vi "Trigger Test.vi"() -> ()   [LabVIEW 2018]
panel:
  in  "Quit":bool
  out "Frames Per Second":dbl
  out "Image":u16[][](graph)
  out "Timestamp":dbl
  out "Error Out":errorcluster {"code" format="%.0x"}
  out "DCAM Version":string
  out "Library Version":string
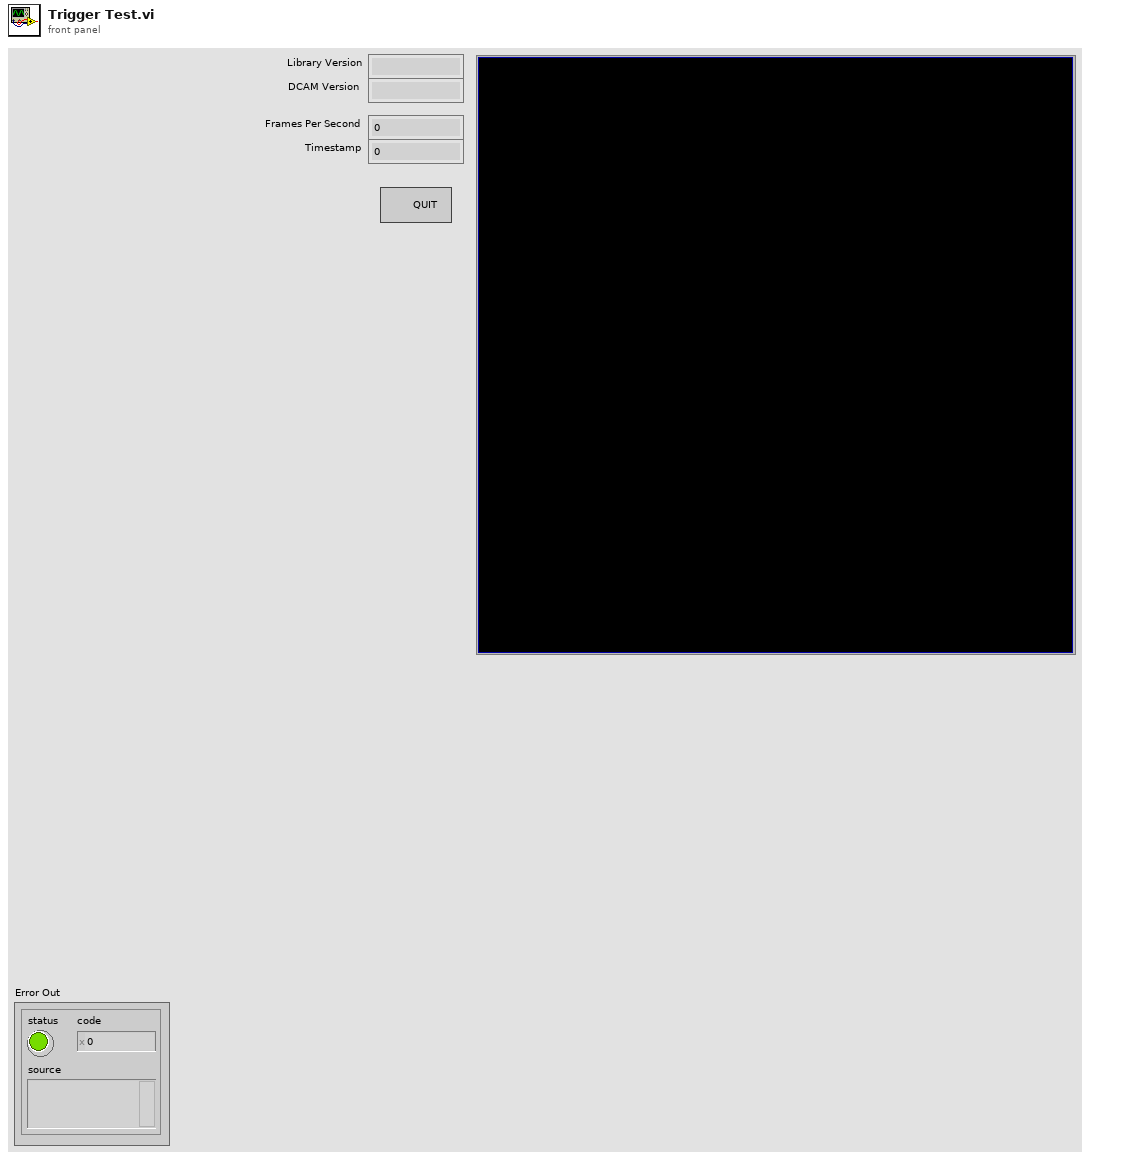
[diagram p1: front panel]
types:
  T1 = cluster{"Capture Library":string, "DCAM-API":string}
  T2 = cluster{"Horizontal Offset":i32, "Vertical Offset":i32, "Horizontal Size":i32, "Vertical Size":i32}
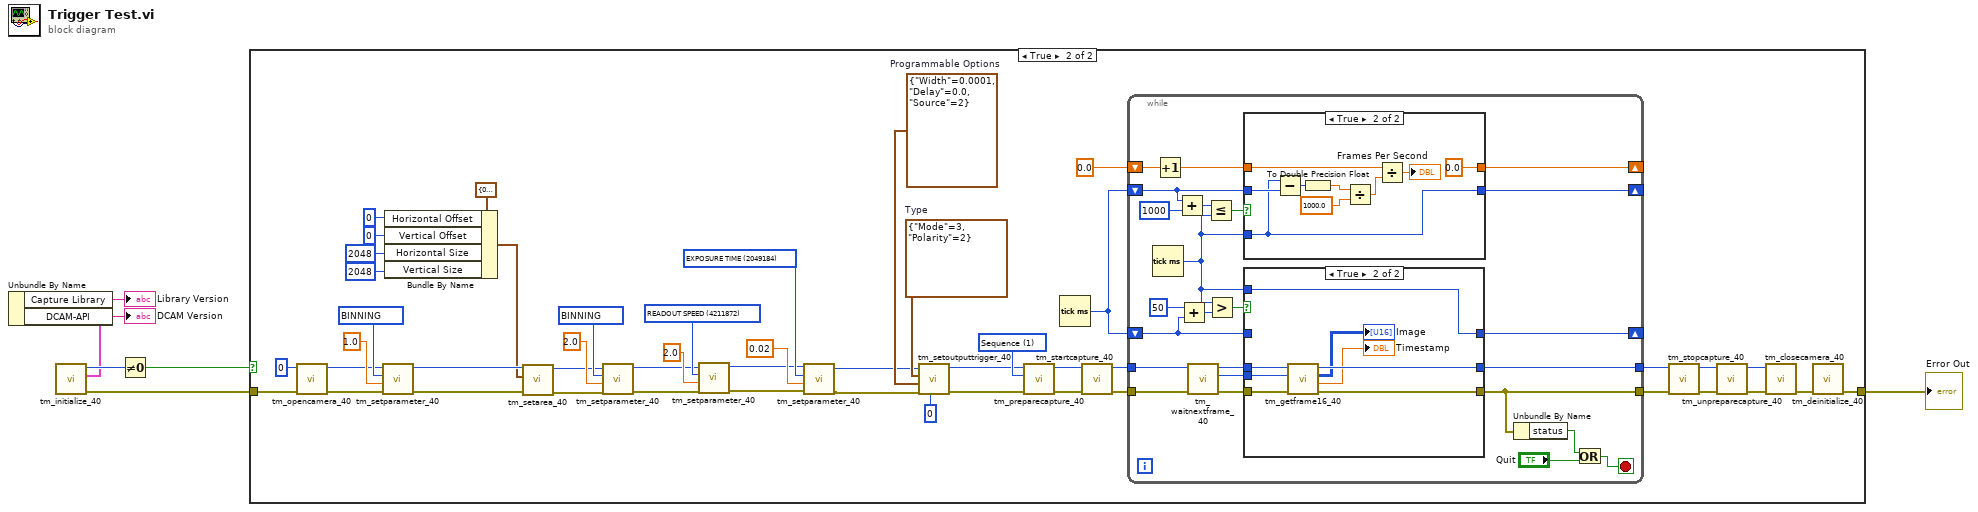
[diagram p0: block diagram]
diagram:
  n1 = call <userlib>:"tm_initialize_40.vi"() -> ("error out"=w2:errorcluster, "Version Info"=w6:T1, "Number Of Cameras"=w7:u32)  [unwired: 8 in, 1 out]
  n2 = Unbundle By Name(w6) -> ("Capture Library"=→"Library Version":string, "DCAM-API"=→"DCAM Version":string)
  n3 = Not Equal To 0?(x=w7) -> (x != 0?=w1:bool)
  n4 = case shown="True" w1 {
    tunnel: w2 -> [w8 w56]
    tunnel: [w8 w40] -> w3
    frame False {
    }
    frame True {
      w11 = cluster{"Width":dbl, "Delay":dbl, "Source":u32} {"Width"=0.0001, "Delay"=0.0, "Source"=2}  # Programmable Options
      w13 = cluster{"Mode":u32, "Polarity":u32} {"Mode"=3, "Polarity"=2}  # Type
      w19 = u32 2049184 items=["SENSOR MODE"=4212128, "READOUT SPEED"=4211872, "READOUT DIRECTION"=4211904, "BIT PER CHANNEL"=4342976, "TRIGGER GLOBAL EXPOSURE"=2049680, "TRIGGER DELAY"=1066480, "SYNC READOUT SYSTEM BLANK"=1066528, "SENSOR COOLER STATUS"=2115280, "EXPOSURE TIME"=2049184, "DEFECT CORRECT MODE"=4670368, "BINNING"=4215968, "TIMING READOUT TIME"=4223904, "INTERNAL FRAME RATE"=4225952, "INTERNAL FRAME INTERVAL"=4225968, "INTERNAL LINE SPEED"=4226000, "INTERNAL LINE INTERVAL"=4226016, "IMAGE WIDTH"=4343200, "IMAGE HEIGHT"=4343216, "IMAGE ROWBYTES"=4343232, "IMAGE FRAMEBYTES"=4343248, "IMAGE PIXEL TYPE"=4343296, "NUMBER OF OUTPUT TRIGGER CONNECTOR"=1852320, "OUTPUT TRIGGER SOURCE[0]"=1852576, "OUTPUT TRIGGER SOURCE[1]"=1852832, "OUTPUT TRIGGER SOURCE[2]"=1853088, "OUTPUT TRIGGER POLARITY[0]"=1852592, "OUTPUT TRIGGER POLARITY[1]"=1852848, "OUTPUT TRIGGER POLARITY[2]"=1853104, "OUTPUT TRIGGER ACTIVE[0]"=1852608, "OUTPUT TRIGGER ACTIVE[1]"=1852864, "OUTPUT TRIGGER ACTIVE[2]"=1853120, "OUTPUT TRIGGER DELAY[0]"=1852624, "OUTPUT TRIGGER DELAY[1]"=1852880, "OUTPUT TRIGGER DELAY[2]"=1853136, "OUTPUT TRIGGER PERIOD[0]"=1852640, "OUTPUT TRIGGER PERIOD[1]"=1852896, "OUTPUT TRIGGER PERIOD[2]"=1853152, "OUTPUT TRIGGER KIND[0]"=1852656, "OUTPUT TRIGGER KIND[1]"=1852912, "OUTPUT TRIGGER KIND[2]"=1853168, "OUTPUT TRIGGER PRE HSYNC COUNT"=1852704] ("Parameter")
      w25 = u32 4215968 items=["SENSOR MODE"=4212128, "READOUT SPEED"=4211872, "READOUT DIRECTION"=4211904, "TRIGGER GLOBAL EXPOSURE"=2049680, "TRIGGER DELAY"=1066480, "INTERNAL TRIGGER HANDLING"=1066496, "SYNC READOUT SYSTEM BLANK"=1066528, "SENSOR TEMPERATURE"=2115232, "SENSOR COOLER STATUS"=2115280, "EXPOSURE TIME"=2049184, "DEFECT CORRECT MODE"=4670368, "BINNING"=4215968, "INTERNAL LINE SPEED"=4226000, "INTERNAL LINE INTERVAL"=4226016, "NUMBER OF OUTPUT TRIGGER CONNECTOR"=1852320, "OUTPUT TRIGGER SOURCE[0]"=1852576, "OUTPUT TRIGGER SOURCE[1]"=1852832, "OUTPUT TRIGGER SOURCE[2]"=1853088, "OUTPUT TRIGGER POLARITY[0]"=1852592, "OUTPUT TRIGGER POLARITY[1]"=1852848, "OUTPUT TRIGGER POLARITY[2]"=1853104, "OUTPUT TRIGGER ACTIVE[0]"=1852608, "OUTPUT TRIGGER ACTIVE[1]"=1852864, "OUTPUT TRIGGER ACTIVE[2]"=1853120, "OUTPUT TRIGGER DELAY[0]"=1852624, "OUTPUT TRIGGER DELAY[1]"=1852880, "OUTPUT TRIGGER DELAY[2]"=1853136, "OUTPUT TRIGGER PERIOD[0]"=1852640, "OUTPUT TRIGGER PERIOD[1]"=1852896, "OUTPUT TRIGGER PERIOD[2]"=1853152, "OUTPUT TRIGGER KIND[0]"=1852656, "OUTPUT TRIGGER KIND[1]"=1852912, "OUTPUT TRIGGER KIND[2]"=1853168, "OUTPUT TRIGGER BASE SENSOR[0]"=1852672, "OUTPUT TRIGGER BASE SENSOR[1]"=1852928, "OUTPUT TRIGGER BASE SENSOR[2]"=1853184, "OUTPUT TRIGGER PRE HSYNC COUNT"=1852704] ("Parameter")
      w37 = u32 4215968 items=["SENSOR MODE"=4212128, "READOUT SPEED"=4211872, "READOUT DIRECTION"=4211904, "TRIGGER GLOBAL EXPOSURE"=2049680, "TRIGGER DELAY"=1066480, "INTERNAL TRIGGER HANDLING"=1066496, "SYNC READOUT SYSTEM BLANK"=1066528, "SENSOR TEMPERATURE"=2115232, "SENSOR COOLER STATUS"=2115280, "EXPOSURE TIME"=2049184, "DEFECT CORRECT MODE"=4670368, "BINNING"=4215968, "INTERNAL LINE SPEED"=4226000, "INTERNAL LINE INTERVAL"=4226016, "NUMBER OF OUTPUT TRIGGER CONNECTOR"=1852320, "OUTPUT TRIGGER SOURCE[0]"=1852576, "OUTPUT TRIGGER SOURCE[1]"=1852832, "OUTPUT TRIGGER SOURCE[2]"=1853088, "OUTPUT TRIGGER POLARITY[0]"=1852592, "OUTPUT TRIGGER POLARITY[1]"=1852848, "OUTPUT TRIGGER POLARITY[2]"=1853104, "OUTPUT TRIGGER ACTIVE[0]"=1852608, "OUTPUT TRIGGER ACTIVE[1]"=1852864, "OUTPUT TRIGGER ACTIVE[2]"=1853120, "OUTPUT TRIGGER DELAY[0]"=1852624, "OUTPUT TRIGGER DELAY[1]"=1852880, "OUTPUT TRIGGER DELAY[2]"=1853136, "OUTPUT TRIGGER PERIOD[0]"=1852640, "OUTPUT TRIGGER PERIOD[1]"=1852896, "OUTPUT TRIGGER PERIOD[2]"=1853152, "OUTPUT TRIGGER KIND[0]"=1852656, "OUTPUT TRIGGER KIND[1]"=1852912, "OUTPUT TRIGGER KIND[2]"=1853168, "OUTPUT TRIGGER BASE SENSOR[0]"=1852672, "OUTPUT TRIGGER BASE SENSOR[1]"=1852928, "OUTPUT TRIGGER BASE SENSOR[2]"=1853184, "OUTPUT TRIGGER PRE HSYNC COUNT"=1852704] ("Parameter")
      w39 = u32 4211872 items=["SENSOR MODE"=4212128, "READOUT SPEED"=4211872, "READOUT DIRECTION"=4211904, "BIT PER CHANNEL"=4342976, "TRIGGER GLOBAL EXPOSURE"=2049680, "TRIGGER DELAY"=1066480, "SYNC READOUT SYSTEM BLANK"=1066528, "SENSOR COOLER STATUS"=2115280, "EXPOSURE TIME"=2049184, "DEFECT CORRECT MODE"=4670368, "BINNING"=4215968, "TIMING READOUT TIME"=4223904, "INTERNAL FRAME RATE"=4225952, "INTERNAL FRAME INTERVAL"=4225968, "INTERNAL LINE SPEED"=4226000, "INTERNAL LINE INTERVAL"=4226016, "IMAGE WIDTH"=4343200, "IMAGE HEIGHT"=4343216, "IMAGE ROWBYTES"=4343232, "IMAGE FRAMEBYTES"=4343248, "IMAGE PIXEL TYPE"=4343296, "NUMBER OF OUTPUT TRIGGER CONNECTOR"=1852320, "OUTPUT TRIGGER SOURCE[0]"=1852576, "OUTPUT TRIGGER SOURCE[1]"=1852832, "OUTPUT TRIGGER SOURCE[2]"=1853088, "OUTPUT TRIGGER POLARITY[0]"=1852592, "OUTPUT TRIGGER POLARITY[1]"=1852848, "OUTPUT TRIGGER POLARITY[2]"=1853104, "OUTPUT TRIGGER ACTIVE[0]"=1852608, "OUTPUT TRIGGER ACTIVE[1]"=1852864, "OUTPUT TRIGGER ACTIVE[2]"=1853120, "OUTPUT TRIGGER DELAY[0]"=1852624, "OUTPUT TRIGGER DELAY[1]"=1852880, "OUTPUT TRIGGER DELAY[2]"=1853136, "OUTPUT TRIGGER PERIOD[0]"=1852640, "OUTPUT TRIGGER PERIOD[1]"=1852896, "OUTPUT TRIGGER PERIOD[2]"=1853152, "OUTPUT TRIGGER KIND[0]"=1852656, "OUTPUT TRIGGER KIND[1]"=1852912, "OUTPUT TRIGGER KIND[2]"=1853168, "OUTPUT TRIGGER PRE HSYNC COUNT"=1852704] ("Parameter")
      w46 = 1 items=["Snap", "Sequence"] ("Capture mode")
      n5 = call <userlib>:"tm_opencamera_40.vi"("error in (no error)"=w56, "Camera Index"=u32 0) -> ("error out"=w34:errorcluster, "Handle out"=w35:u32)  [unwired: 7 in, 1 out]
      n6 = call <userlib>:"tm_setparameter_40.vi"("error in (no error)"=w34, "Value in"=1.0, "Parameter"=w37, "Handle in"=w35) -> ("error out"=w32:errorcluster, "Handle out"=w33:u32)  [unwired: 6 in]
      n7 = Bundle By Name(cluster=T2 {"Horizontal Offset"=0, "Vertical Offset"=0, "Horizontal Size"=0, "Vertical Size"=0} ("Sub Region"), "Horizontal Offset"=0, "Vertical Offset"=0, "Horizontal Size"=2048, "Vertical Size"=2048) -> (w27:T2)
      n8 = call <userlib>:"tm_setarea_40.vi"("error in (no error)"=w32, "Sub Region"=w27, "Handle in"=w33) -> ("error out"=w22:errorcluster, "Handle out"=w23:u32)  [unwired: 7 in]
      n9 = call <userlib>:"tm_setparameter_40.vi"("error in (no error)"=w22, "Value in"=2.0, "Parameter"=w25, "Handle in"=w23) -> ("error out"=w20:errorcluster, "Handle out"=w21:u32)  [unwired: 6 in]
      n10 = call <userlib>:"tm_setparameter_40.vi"("error in (no error)"=w20, "Value in"=2.0, "Parameter"=w39, "Handle in"=w21) -> ("error out"=w16:errorcluster, "Handle out"=w17:u32)  [unwired: 6 in]
      n11 = call <userlib>:"tm_setparameter_40.vi"("error in (no error)"=w16, "Value in"=0.02, "Parameter"=w19, "Handle in"=w17) -> ("error out"=w9:errorcluster, "Handle out"=w10:u32)  [unwired: 6 in]
      n12 = call <userlib>:"tm_setoutputtrigger_40.vi"("Port"=0, "error in (no error)"=w9, "Programmable Options"=w11, "Type"=w13, "Handle in"=w10) -> ("error out"=w14:errorcluster, "Handle out"=w15:u32)  [unwired: 5 in]
      n13 = call <userlib>:"tm_preparecapture_40.vi"("error in (no error)"=w14, "Capture mode"=w46, "Handle in"=w15) -> ("error out"=w44:errorcluster, "Handle out"=w45:u32)  [unwired: 5 in, 2 out]
      n14 = Tick Count (ms)() -> (millisecond timer value=w42:u32)
      n15 = call <userlib>:"tm_startcapture_40.vi"("error in (no error)"=w44, "Handle in"=w45) -> ("error out"=w47:errorcluster, "Handle out"=w48:u32)  [unwired: 8 in]
      n16 = while {
        tunnel: [w59] -> w51
        tunnel: [w60] -> w52
        tunnel: w48 -> [w77]
        tunnel: w47 -> [w78]
        shift-right: [w75] -> _
        shift-left: w42 -> [w72]
        shift-right: [w76] -> _
        shift-left: 0.0 -> [w69]
        shift-right: [w58] -> _
        shift-left: w42 -> [w61]
        stop <- w57 stop-if-true
        n17 = Tick Count (ms)() -> (millisecond timer value=w62:u32)
        n18 = Increment(x=w69) -> (x+1=w70:dbl)
        n19 = Add(x=w72, y=u32 1000) -> (x+y=w74:u32)
        n20 = Add(x=u32 50, y=w61) -> (x+y=w64:u32)
        n21 = call <userlib>:"tm_waitnextframe_40.vi"("error in (no error)"=w78, "Handle in"=w77) -> ("error out"=w67:errorcluster, "Frame Index"=w66:i32, "Handle out"=w68:u32)  [unwired: 6 in, 1 out]
        n22 = Less Or Equal?(x=w74, y=w62) -> (x <= y?=w71:bool)
        n23 = Greater?(x=w62, y=w64) -> (0:w63:bool)
        n24 = case shown="True" w71 {
          tunnel: w72 -> [w93 w96]
          tunnel: [w93 w94] -> w75
          tunnel: w70 -> [w92 w100]
          tunnel: w62 -> [_ w94]
          tunnel: [w92 0.0] -> w76
          frame False {
          }
          frame True {
            n25 = Subtract(x=w94, y=w96) -> (x-y=w95:u32)
            n26 = To Double Precision Float(number=w95) -> (double precision float=w102:dbl)
            n27 = Divide(x=w102, y=1000.0) -> (x/y=w99:dbl)
            n28 = Divide(x=w100, y=w99) -> (x/y=→"Frames Per Second":dbl)
          }
        }
        n29 = case shown="True" w63 {
          tunnel: w68 -> [w83 w91]
          tunnel: w67 -> [w82 w90]
          tunnel: w66 -> [_ w84]
          tunnel: w61 -> [w81 _]
          tunnel: w62 -> [_ w89]
          tunnel: [w83 w87] -> w59
          tunnel: [w82 w88] -> w60
          tunnel: [w81 w89] -> w58
          frame False {
          }
          frame True {
            n30 = call <userlib>:"tm_getframe16_40.vi"("error in (no error)"=w90, "Frame Index"=w84, "Handle in"=w91) -> ("error out"=w88:errorcluster, "Timestamp"=→"Timestamp":dbl, "Data"=→"Image":u16[][], "Handle out"=w87:u32)  [unwired: 5 in]
          }
        }
        n31 = Unbundle By Name(w60) -> ("status"=w80:bool)
        n32 = Or(x=w80, y="Quit") -> (x .or. y?=w57:bool)
      }
      n33 = call <userlib>:"tm_stopcapture_40.vi"("error in (no error)"=w52, "Handle in"=w51) -> ("error out"=w49:errorcluster, "Handle out"=w50:u32)  [unwired: 8 in]
      n34 = call <userlib>:"tm_unpreparecapture_40.vi"("error in (no error)"=w49, "Handle in"=w50) -> ("error out"=w54:errorcluster, "Handle out"=w53:u32)  [unwired: 8 in]
      n35 = call <userlib>:"tm_closecamera_40.vi"("error in (no error)"=w54, "Handle in"=w53) -> ("error out"=w41:errorcluster)  [unwired: 9 in]
      n36 = call <userlib>:"tm_deinitialize_40.vi"("error in (no error)"=w41) -> ("error out"=w40:errorcluster)  [unwired: 10 in]
    }
  }
  "Error Out" <- w3
